vi "Write Fill Style.vi"(5 "Fill Style":i32, 9 "Slide in":refnum<class "Slide.lvclass">) -> (3 "Slide out":refnum<class "Slide.lvclass">)   [LabVIEW 2014, in "Raspberry Pi Compatible Compiler for LabVIEW.lvlib" / "Slide.lvclass"]
uses:
  Slide.lvclass
  Slide.lvclass/Slide.ctl
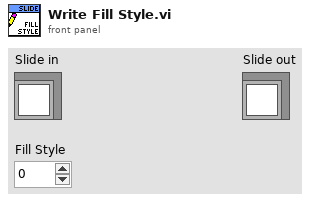
[diagram p1: front panel]
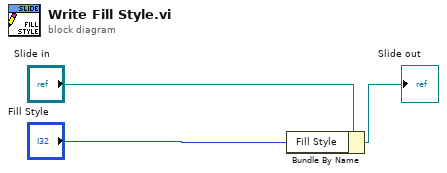
[diagram p0: block diagram]
diagram:
  n1 = Bundle By Name(cluster="Slide in", "Fill Style"="Fill Style") -> (→"Slide out":refnum<class "Slide.lvclass">)
